vi "TEST MENU RING CONTROLS.vi"() -> ()   [LabVIEW 2023]
panel:
  out "Ring 2":dbl(ring) items=["TEST 2"=-0.39, "TEST 1"=0.53]
  in  "Ring":dbl(ring) format="%.3f" items=["this is test 2 that should give the value -0.390"=-0.39, "TEST 1"=0.53]
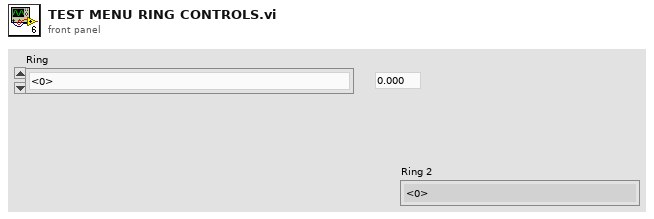
[diagram p1: front panel]
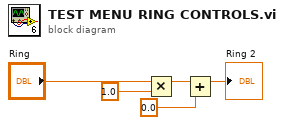
[diagram p0: block diagram]
diagram:
  n1 = Multiply(x="Ring", y=1.0) -> (x*y=w4:dbl)
  n2 = Add(x=w4, y=0.0) -> (x+y=→"Ring 2":dbl)
